vi "FPGA_main.vi"() -> ()   [LabVIEW 2020]
uses:
  <vilib>/eio/EIONode/EIONode.xnode
  <vilib>/rvi/eio/common/nirviEmuTemplateMethod_errors.vi
  <vilib>/platform/TimedLoop/XDataNode/XDataNode.xnode
  <vilib>/Platform/TimedLoop/XDataNode/nitl_modes.ctl
  <vilib>/Platform/TimedLoop/XDataNode/XDNodeRunTimeDep.lvlib
  <vilib>/Platform/TimedLoop/XDataNode/wakeup.ctl
  <vilib>/Platform/TimedLoop/XDataNode/timing_clust.ctl
  <vilib>/rvi/DataTransferAndStorage/Container/XNode/niFpgaContainer.xnode
  <vilib>/rvi/interface/RandomDataEmulation/nirviRandomDataFpgaReadWriteTemplate.vi
  <vilib>/eio/EIOPropertyNode/EIOPropertyNode.xnode
  <vilib>/rvi/eio/common/nirviEmuTemplatePropertyGet_errors.vi
  <vilib>/rvi/eio/common/nirviEmuTemplatePropertyGet_noerrors.vi
  <vilib>/rvi/eio/common/nirviEmuTemplatePropertySet_errors.vi
  <vilib>/rvi/eio/common/nirviEmuTemplatePropertySet_noerrors.vi
  <vilib>/eio/EIOMethodNode/EIOMethodNode.xnode
  <vilib>/LabVIEW Targets/FPGA/cRIO/shared/nicrio_ModuleControls/nicrio_cRIO-9775_ContinuousDataRates4ChansRing.ctl
  <vilib>/LabVIEW Targets/FPGA/cRIO/shared/nicrio_ModuleControls/nicrio_BasicConversionTime.ctl
panel:
  in  "error in":errorcluster
  in  "Enable Low Pass Filter":T1
  out "FPGA Error Out":errorcluster
  in  "Timing Mode":T2
  in  "Continuous Data Rate":T3=20 items=["1.000 MS/s (NI 9775)"=20, "833.333 KS/s (NI 9775)"=24, "714.286 KS/s (NI 9775)"=28, "625.000 KS/s (NI 9775)"=32, "555.556 KS/s (NI 9775)"=36, "500.000 KS/s (NI 9775)"=40, "454.545 KS/s (NI 9775)"=44, "416.667 KS/s (NI 9775)"=48, "384.615 KS/s (NI 9775)"=52, "357.143 KS/s (NI 9775)"=56, "333.333 KS/s (NI 9775)"=60, "312.500 KS/s (NI 9775)"=64, "294.118 KS/s (NI 9775)"=68, "277.778 KS/s (NI 9775)"=72, "263.158 KS/s (NI 9775)"=76, "250.000 KS/s (NI 9775)"=80, "238.095 KS/s (NI 9775)"=84, "227.273 KS/s (NI 9775)"=88, "217.391 KS/s (NI 9775)"=92, "208.333 KS/s (NI 9775)"=96, "200.000 KS/s (NI 9775)"=100, "192.308 KS/s (NI 9775)"=104, "185.185 KS/s (NI 9775)"=108, "178.571 KS/s (NI 9775)"=112, "172.414 KS/s (NI 9775)"=116, "166.667 KS/s (NI 9775)"=120, "161.290 KS/s (NI 9775)"=124, "156.250 KS/s (NI 9775)"=128, "151.515 KS/s (NI 9775)"=132, "147.059 KS/s (NI 9775)"=136, "142.857 KS/s (NI 9775)"=140, "138.889 KS/s (NI 9775)"=144, "135.135 KS/s (NI 9775)"=148, "131.579 KS/s (NI 9775)"=152, "128.205 KS/s (NI 9775)"=156, "125.000 KS/s (NI 9775)"=160, "121.951 KS/s (NI 9775)"=164, "119.048 KS/s (NI 9775)"=168, "116.279 KS/s (NI 9775)"=172, "113.636 KS/s (NI 9775)"=176, "111.111 KS/s (NI 9775)"=180, "108.696 KS/s (NI 9775)"=184, "106.383 KS/s (NI 9775)"=188, "104.167 KS/s (NI 9775)"=192, "102.041 KS/s (NI 9775)"=196, "100.000 KS/s (NI 9775)"=200, "50.000 KS/s (NI 9775)"=400, "33.333 KS/s (NI 9775)"=600, "25.000 KS/s (NI 9775)"=800, "20.000 KS/s (NI 9775)"=1000, "16.667 KS/s (NI 9775)"=1200, "14.286 KS/s (NI 9775)"=1400, "12.500 KS/s (NI 9775)"=1600, "11.111 KS/s (NI 9775)"=1800, "10.000 KS/s (NI 9775)"=2000, "9.091 KS/s (NI 9775)"=2200, "8.333 KS/s (NI 9775)"=2400, "7.692 KS/s (NI 9775)"=2600, "7.143 KS/s (NI 9775)"=2800, "6.667 KS/s (NI 9775)"=3000, "6.250 KS/s (NI 9775)"=3200, "5.882 KS/s (NI 9775)"=3400, "5.556 KS/s (NI 9775)"=3600, "5.000 KS/s (NI 9775)"=4000, "4.762 KS/s (NI 9775)"=4200, "4.545 KS/s (NI 9775)"=4400, "4.348 KS/s (NI 9775)"=4600, "4.167 KS/s (NI 9775)"=4800, "4.000 KS/s (NI 9775)"=5000, "3.846 KS/s (NI 9775)"=5200, "3.571 KS/s (NI 9775)"=5600, "3.333 KS/s (NI 9775)"=6000, "3.125 KS/s (NI 9775)"=6400, "2.941 KS/s (NI 9775)"=6800, "2.778 KS/s (NI 9775)"=7200, "2.632 KS/s (NI 9775)"=7600, "2.500 KS/s (NI 9775)"=8000, "2.381 KS/s (NI 9775)"=8400, "2.273 KS/s (NI 9775)"=8800, "2.174 KS/s (NI 9775)"=9200, "2.083 KS/s (NI 9775)"=9600, "2.000 KS/s (NI 9775)"=10000, "1.923 KS/s (NI 9775)"=10400, "1.852 KS/s (NI 9775)"=10800, "1.786 KS/s (NI 9775)"=11200, "1.724 KS/s (NI 9775)"=11600, "1.667 KS/s (NI 9775)"=12000, "1.613 KS/s (NI 9775)"=12400, "1.563 KS/s (NI 9775)"=12800, "1.515 KS/s (NI 9775)"=13200, "1.471 KS/s (NI 9775)"=13600, "1.429 KS/s (NI 9775)"=14000, "1.389 KS/s (NI 9775)"=14400, "1.351 KS/s (NI 9775)"=14800, "1.316 KS/s (NI 9775)"=15200, "1.282 KS/s (NI 9775)"=15600, "1.250 KS/s (NI 9775)"=16000, "1.220 KS/s (NI 9775)"=16400, "1.190 KS/s (NI 9775)"=16800, "1.163 KS/s (NI 9775)"=17200, "1.136 KS/s (NI 9775)"=17600, "1.111 KS/s (NI 9775)"=18000, "1.087 KS/s (NI 9775)"=18400, "1.064 KS/s (NI 9775)"=18800, "1.042 KS/s (NI 9775)"=19200, "1.020 KS/s (NI 9775)"=19600, "1.000 KS/s (NI 9775)"=20000, "0.980 KS/s (NI 9775)"=20400, "0.962 KS/s (NI 9775)"=20800, "0.943 KS/s (NI 9775)"=21200, "0.926 KS/s (NI 9775)"=21600, "0.909 KS/s (NI 9775)"=22000, "0.893 KS/s (NI 9775)"=22400, "0.877 KS/s (NI 9775)"=22800, "0.862 KS/s (NI 9775)"=23200, "0.847 KS/s (NI 9775)"=23600, "0.833 KS/s (NI 9775)"=24000, "0.820 KS/s (NI 9775)"=24400, "0.806 KS/s (NI 9775)"=24800, "0.794 KS/s (NI 9775)"=25200, "0.781 KS/s (NI 9775)"=25600, "0.694 KS/s (NI 9775)"=28800, "0.625 KS/s (NI 9775)"=32000, "0.568 KS/s (NI 9775)"=35200, "0.521 KS/s (NI 9775)"=38400, "0.446 KS/s (NI 9775)"=44800, "0.391 KS/s (NI 9775)"=51200, "0.347 KS/s (NI 9775)"=57600, "0.313 KS/s (NI 9775)"=64000]
  out "Data FIFO Full":bool
  out "Count Timouts":i32
  out "Bin Size \n(ticks)":u32
  in  "Stream counts?":bool
  out "Overflow":bool
  in  "Bin Size(uSec)":u32=1 caption="Count(uSec)"
  in  "Reset Photon Count":bool
  in  "Type Counter":enum16{"Falling Edge", "Rising Edge"}(ring)
  out "Total Counts":i32
  # "Photon counting. Single cycle time loop"
  # "User Control of digital output"
  # "Binning and streaming binned Total Count"
  # "Streaming Analog Input Data"
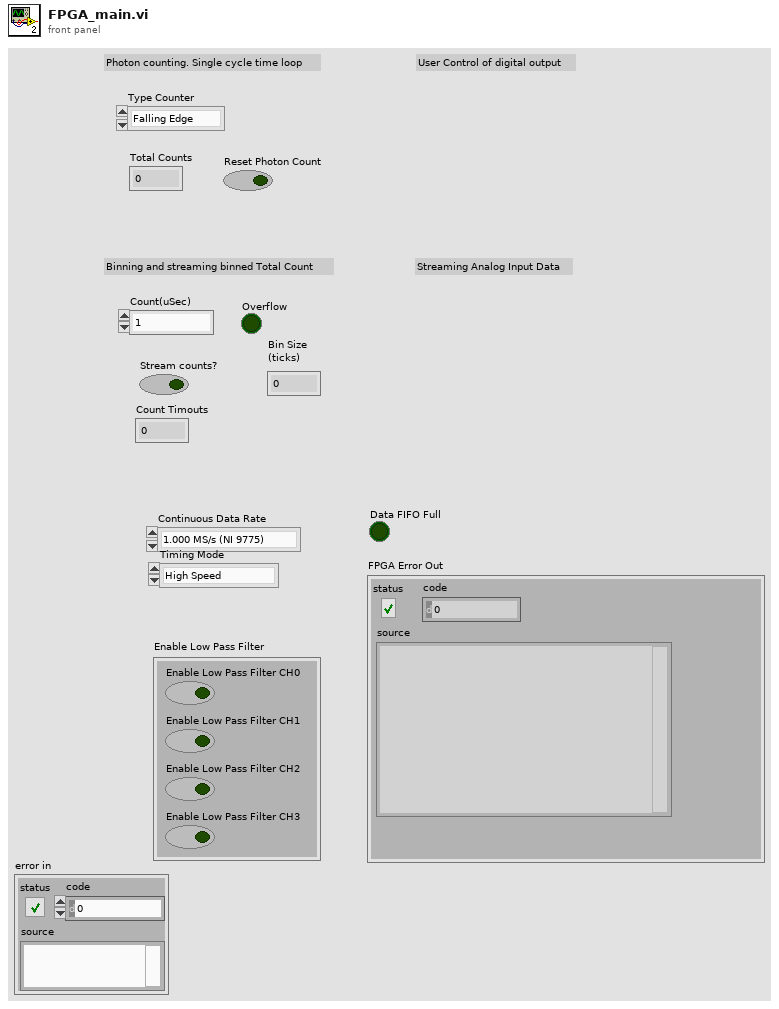
[diagram p1: front panel]
types:
  T1 = cluster{"Enable Low Pass Filter CH1":bool, "Enable Low Pass Filter CH2":bool, "Enable Low Pass Filter CH3":bool, "Enable Low Pass Filter CH0":bool}
  T2 = typedef "nicrio_BasicConversionTime.ctl" = enum8{"High Speed", "High Resolution"}
  T3 = typedef "nicrio_cRIO-9775_ContinuousDataRates4ChansRing.ctl" = u16
  T4 = typedef "XDNodeRunTimeDep.lvlib/timing_clust.ctl" = cluster{"Expected End [f-1]":u64, "Actual End [f-1]":u64, "Finished Late? [f-1]":bool, "Expected End [i-1]":u64, "Actual End [i-1]":u64, "Finished Late? [i-1]":bool, "Expected Start [i]":u64, "Actual Start [i]":u64, "Expected Start [f]":u64, "Actual Start [f]":u64, "Source Name":string, "Structure Name":string, "Period":i64, "Deadline":i64, "Offset":i64, "Start":i64, "Priority":i32, "Timeout":i32, "Mode":T5, "Wakeup Reason":T6, "Error":errorcluster, "Source Type":string, "Secondary Source Type":string, "Global End Time":u64, "Global Start Time":u64, "Frame Duration":u64, "Iteration Duration":u64, "Assigned CPU":i32, "I/O Scan Engine Mode":u32}
  T5 = typedef "XDNodeRunTimeDep.lvlib/nitl_modes.ctl" = enum32{"No Change", "Process missed periods, maintain original phase", "Discard missed periods, maintain original phase", "Process missed periods, ignore original phase", "Discard missed periods, ignore original phase"}
  T6 = typedef "XDNodeRunTimeDep.lvlib/wakeup.ctl" = enum32{"Normal", "Aborted", "Asynchronous wakeup", "Timing source error", "Timed loop error", "Timeout"}
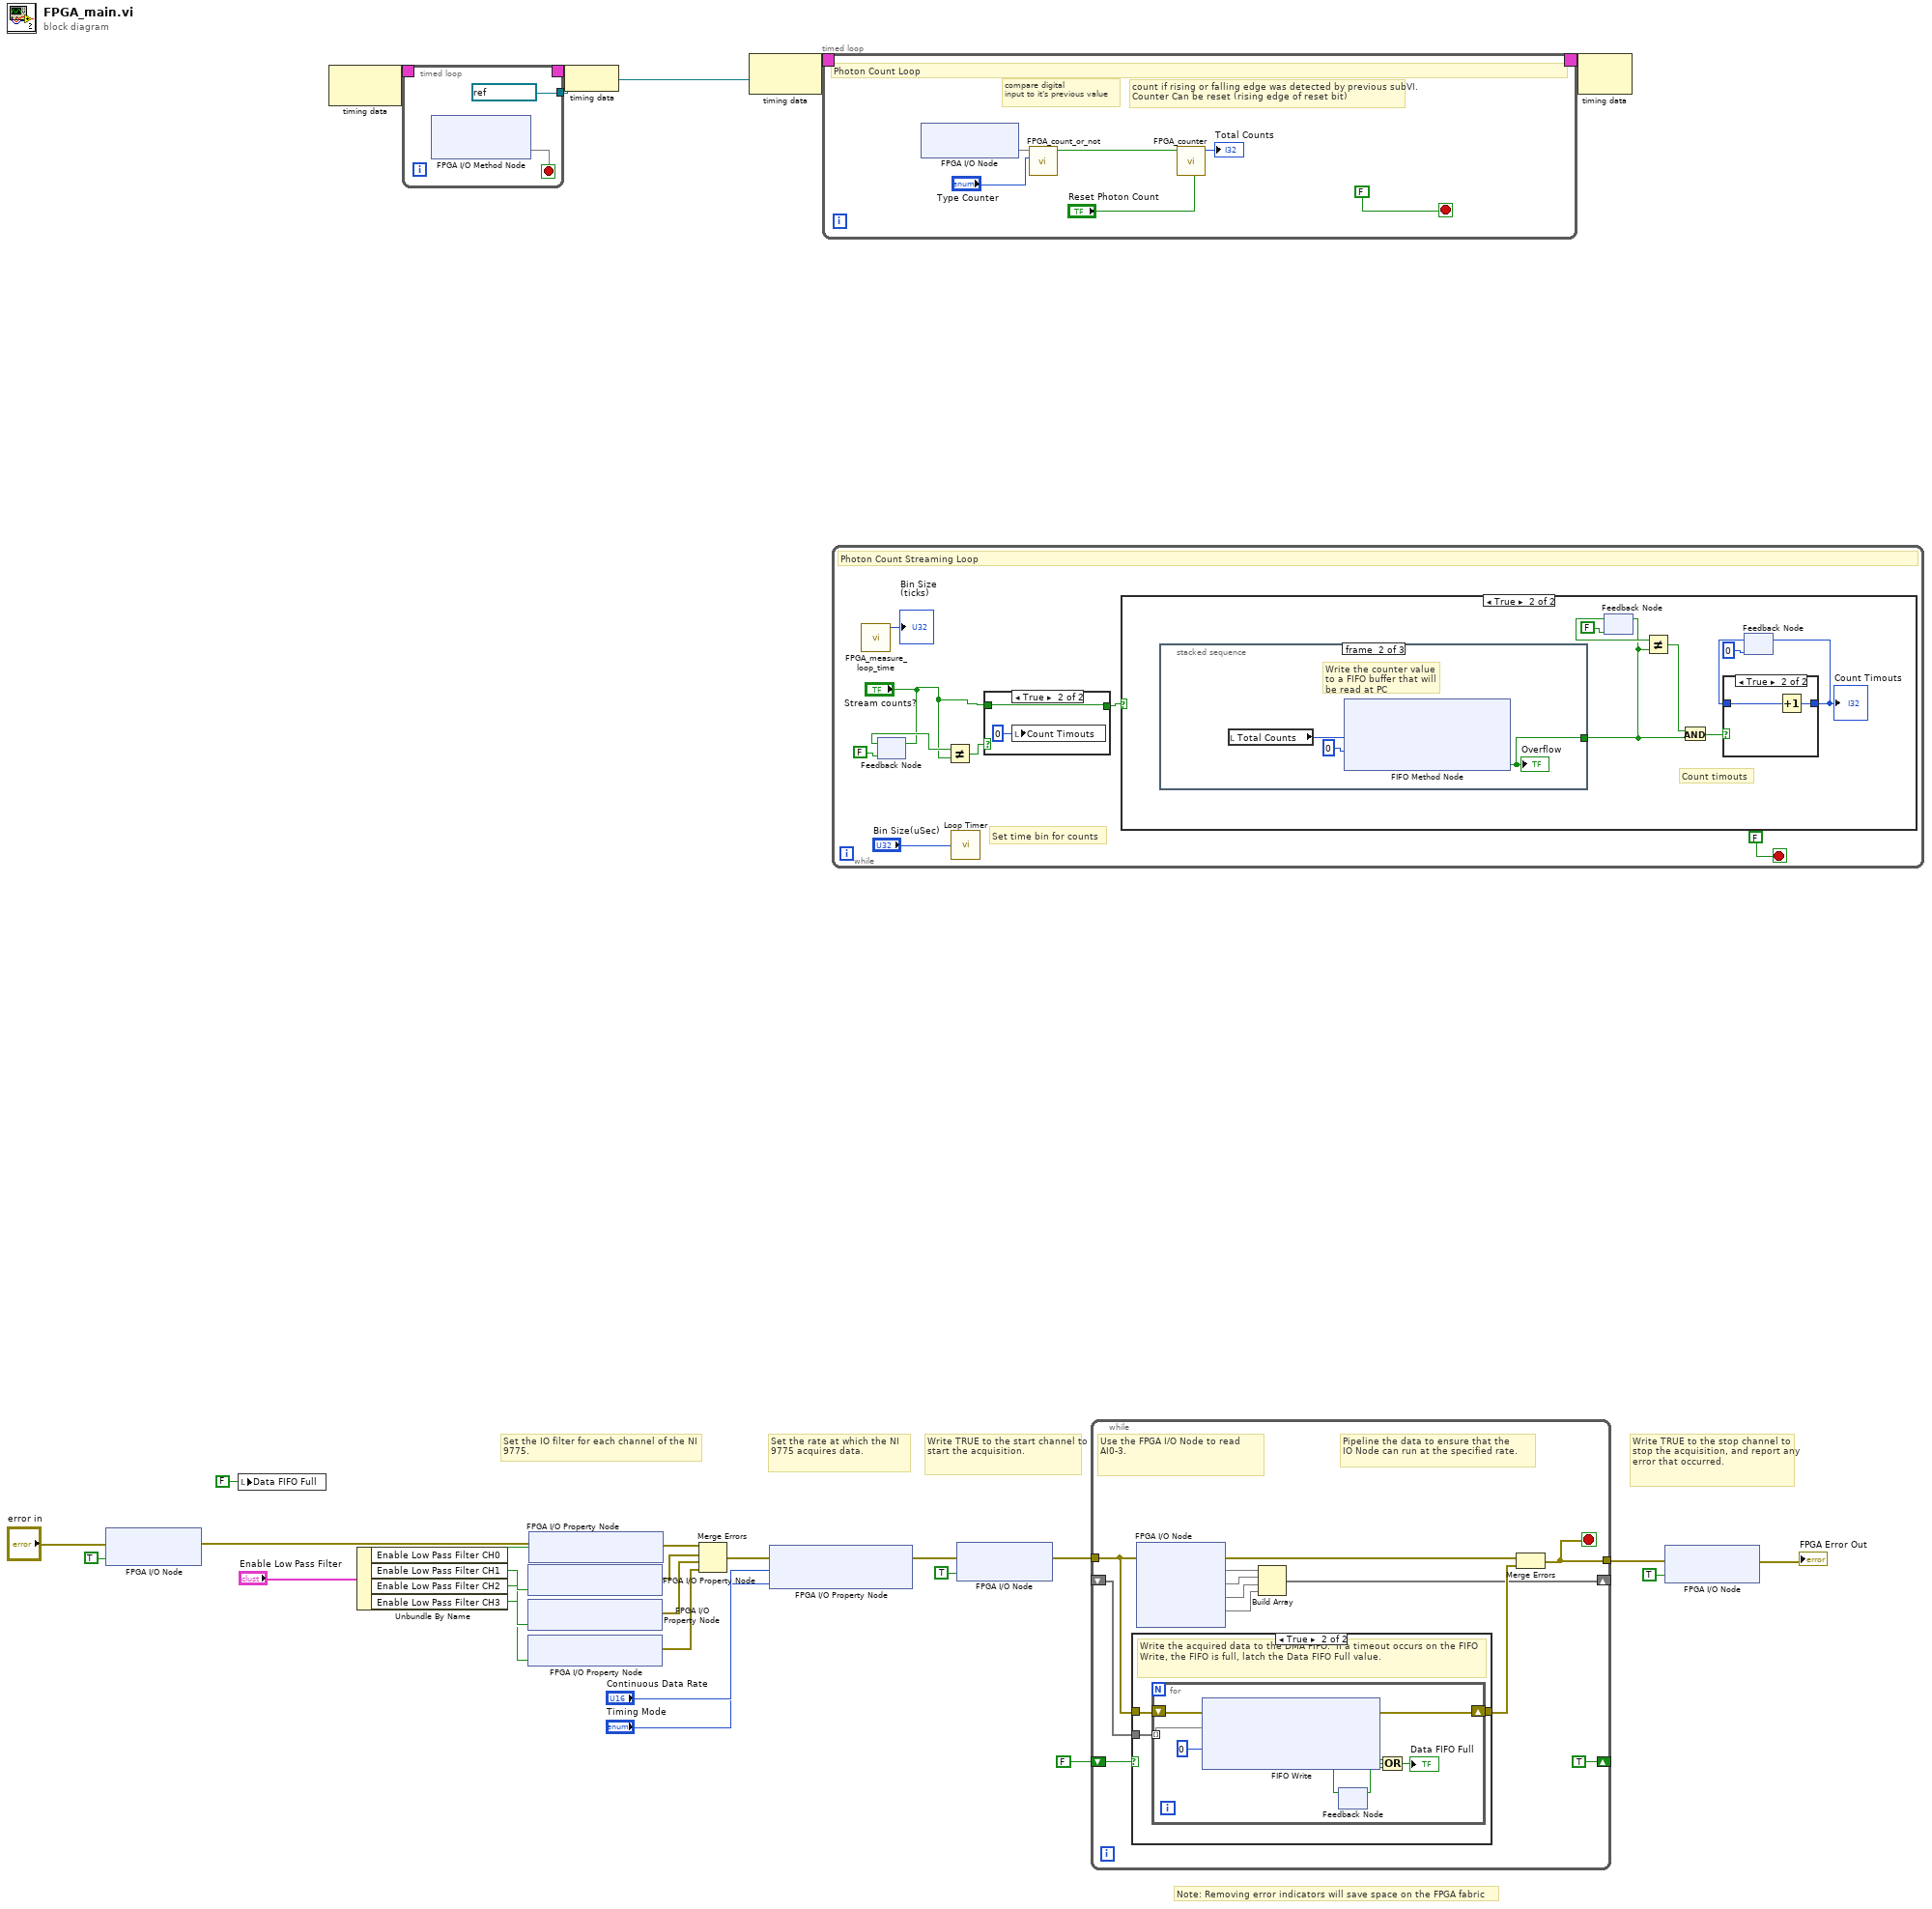
[diagram p0: block diagram]
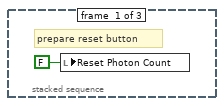
[diagram p6: hidden frame]
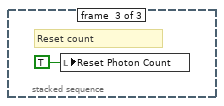
[diagram p7: hidden frame]
diagram:
  # "Write TRUE to the stop channel to stop the acquisition, and report any error that occurred."
  # "Note: Removing error indicators will save space on the FPGA fabric"
  # "Write TRUE to the start channel to start the acquisition."
  # "Set the rate at which the NI 9775 acquires data."
  # "Set the IO filter for each channel of the NI 9775."
  n1 = xnode "FPGA I/O Node"("error in"="error in", "Mod1/Stop"=TRUE) -> ("error out"=w3:errorcluster)  [unwired: 1 in, 1 out]
  n2 = local write "Data FIFO Full"(FALSE ("Data FIFO Full")) -> ()
  n3 = node-c288() -> (w25:T4)  [unwired: 1 in]
  n4 = Unbundle By Name("Enable Low Pass Filter") -> ("Enable Low Pass Filter CH0"=w8:bool, "Enable Low Pass Filter CH1"=w7:bool, "Enable Low Pass Filter CH2"=w6:bool, "Enable Low Pass Filter CH3"=w5:bool)
  n5 = timed-loop {
    tunnel: [refnum<k21> "120MHz" ("Source Name")] -> w26
    timing: w25 -> [_]
    timing-out: [_] -> w24
    stop <- w29 stop-if-true
    n6 = xnode "FPGA I/O Method Node"() -> ("Ready"=w29)  [unwired: 1 in, 1 out]
  }
  n7 = xnode "FPGA I/O Property Node"("Enable Analog Filter"=w7) -> ("error out"=w17:errorcluster)  [unwired: 2 in, 1 out]
  n8 = xnode "FPGA I/O Property Node"("Enable Analog Filter"=w6) -> ("error out"=w16:errorcluster)  [unwired: 2 in, 1 out]
  n9 = xnode "FPGA I/O Property Node"("Enable Analog Filter"=w5) -> ("error out"=w15:errorcluster)  [unwired: 2 in, 1 out]
  n10 = xnode "FPGA I/O Property Node"("error in"=w3, "Enable Analog Filter"=w8) -> ("error out"=w19:errorcluster)  [unwired: 1 in, 1 out]
  n11 = node-c288(w24) -> ()
  n12 = Merge Errors(w19, w17, w16, w15) -> (w18:errorcluster)
  n13 = node-c288(w26) -> (w28:T4)
  n14 = xnode "FPGA I/O Property Node"("error in"=w18, "Continuous Data Rate"="Continuous Data Rate", "Timing Mode"="Timing Mode") -> ("error out"=w11:errorcluster)  [unwired: 1 in, 1 out]
  n15 = timed-loop {
    timing: w28 -> [_]
    timing-out: [_] -> w27
    stop <- FALSE stop-if-true
    # "count if rising or falling edge was detected by previous subVI. Counter Can be reset (rising edge of reset bit)"
    # "compare digital\ninput to it's previous value"
    # "Photon Count Loop"
    n16 = xnode "FPGA I/O Node"() -> ("Mod2/DIO0"=w36)  [unwired: 1 in, 1 out]
    n17 = call "FPGA_count_or_not.vi"("Type Counter"="Type Counter", "Countable"=w36) -> ("Count or Not?"=w37:bool)  [unwired: 9 in]
    n18 = call "FPGA_counter.vi"("Count or Not?"=w37, "Reset Photon Count"="Reset Photon Count") -> ("Total Count"=→"Total Counts":u8)  [unwired: 8 in]
  }
  n19 = while {
    stop <- FALSE stop-if-true
    # "Set time bin for counts"
    # "Photon Count Streaming Loop"
    n20 = call "FPGA_measure_loop_time.vi"() -> ("Numeric"=→"Bin Size \n(ticks)":u32)  [unwired: 11 in]
    n21 = feedback #1(FALSE) -> (w44:bool)
    n22 = feedback-in #1("Stream counts?") -> ()
    n23 = Not Equal?(x=w44, y="Stream counts?") -> (x != y?=w43:bool)
    n24 = call "Loop Timer"("Count(uSec)"="Bin Size(uSec)") -> ()  [unwired: 1 out]
    n25 = case shown="True" w43 {
      tunnel: "Stream counts?" -> [w49 w50]
      tunnel: [w49 w50] -> w41
      frame False {
      }
      frame True {
        n26 = local write "Count Timouts"(0 ("Count Timouts")) -> ()
      }
    }
    n27 = case shown="True" w41 {
      frame False {
      }
      frame True {
        # "Count timouts"
        n28 = stacked-sequence {
          tunnel: [_ w64 _] -> w52
          frame #0 {
            # "prepare reset button"
            n29 = local write "Reset Photon Count"(FALSE) -> ()
          }
          frame #1 {
            # "Write the counter value to a FIFO buffer that will be read at PC"
            n30 = local read "Total Counts"() -> (w66:i32)
            n31 = xnode ("FIFO Method Node")("Element"=w66, "Timeout"=0) -> ("Timed Out?"=w64:bool)  [unwired: 1 in, 1 out]
            "Overflow" <- w64
          }
          frame #2 {
            # "Reset count"
            n32 = local write "Reset Photon Count"(TRUE) -> ()
          }
        }
        n33 = feedback #2(FALSE) -> (w55:bool)
        n34 = feedback-in #2(w52) -> ()
        n35 = Not Equal?(x=w55, y=w52) -> (x != y?=w54:bool)
        n36 = And(x=w54, y=w52) -> (x .and. y?=w53:bool)
        n37 = feedback #3(0 ("Timeout")) -> (w58:i32)
        n38 = case shown="True" w53 {
          tunnel: w58 -> [w60 w62]
          tunnel: [w60 w61] -> w57
          frame False {
          }
          frame True {
            n39 = Increment(x=w62) -> (x+1=w61:i32)
          }
        }
        "Count Timouts" <- w57
        n40 = feedback-in #3(w57) -> ()
      }
    }
  }
  n41 = xnode "FPGA I/O Node"("error in"=w11, "Mod1/Start"=TRUE) -> ("error out"=w21:errorcluster)  [unwired: 1 in, 1 out]
  n42 = while {
    tunnel: w21 -> [w71]
    tunnel: [w73] -> w23
    shift-right: [TRUE] -> _
    shift-left: FALSE -> [w75]
    shift-right: [w70] -> _
    shift-left: _ -> [w69]
    stop <- w73 stop-if-true
    # "Pipeline the data to ensure that the \nIO Node can run at the specified rate."
    # "Use the FPGA I/O Node to read \nAI0-3."
    n43 = case shown="True" w75 {
      tunnel: [w80 w83] -> w72
      tunnel: w71 -> [w80 w82]
      tunnel: w69 -> [_ w81]
      frame False {
        # "On the initial iteration of the loop we do not put data in the FIFO."
      }
      frame True {
        # "Write the acquired data to the DMA FIFO.  If a timeout occurs on the FIFO Write, the FIFO is full, latch the Data FIFO Full value."
        n44 = for {
          tunnel: w81 -> [w84] mode=indexing
          shift-right: [w85] -> w83
          shift-left: w82 -> [w86]
          n45 = xnode ("FIFO Write")("Element"=w84, "Timeout"=0 ("Timeout (-1 for no timeout)"), "error in (no error)"=w86) -> ("Timed Out?"=w88:bool, "error out"=w85:errorcluster)  [unwired: 1 in, 1 out]
          n46 = feedback #4() -> (w89:bool)  [unwired: 1 out]
          n47 = Or(x=w88, y=w89) -> (x .or. y?=w90:bool)
          "Data FIFO Full" <- w90
          n48 = feedback-in #4(w90) -> ()
        }
      }
    }
    n49 = xnode "FPGA I/O Node"("error in"=w71) -> ("error out"=w74:errorcluster, "Mod1/AI0"=w79, "Mod1/AI1"=w78, "Mod1/AI2"=w77, "Mod1/AI3"=w76)  [unwired: 4 in, 4 out]
    n50 = Build Array(w79, w78, w77, w76) -> (w70:void[])
    n51 = Merge Errors(w74, w72) -> (w73:errorcluster)
  }
  n52 = node-c288(w27) -> ()  [unwired: 1 out]
  n53 = xnode "FPGA I/O Node"("error in"=w23, "Mod1/Stop"=TRUE) -> ("error out"=→"FPGA Error Out":errorcluster)  [unwired: 1 in, 1 out]
